vi "onStop.vi"(8 "error in (no error)":errorcluster, 11 "Client in":refnum<class "Client.lvclass">) -> (0 "error out":errorcluster, 3 "Client out":refnum<class "Client.lvclass">)   [LabVIEW 2013, in "MQTT Server.lvlib" / "Client.lvclass"]
uses:
  Client.lvclass
  MQTT_Base/MQTT_Base.lvclass
  Client.lvclass/Client.ctl
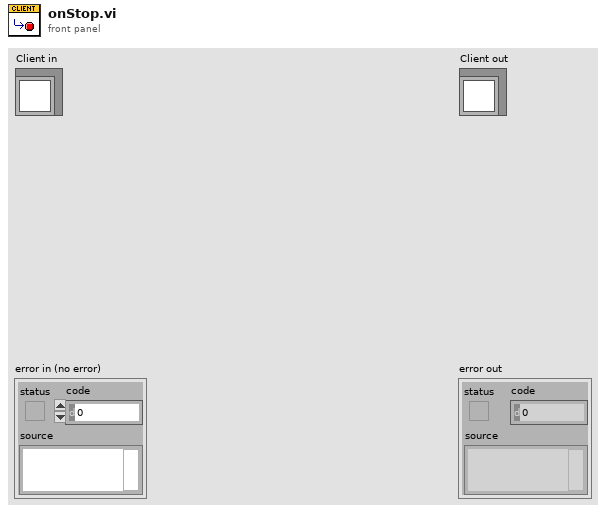
[diagram p1: front panel]
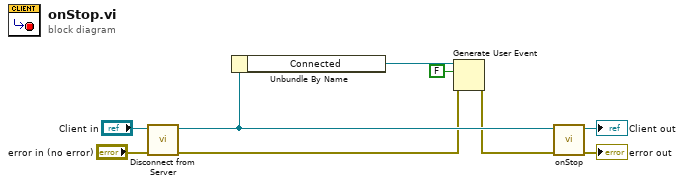
[diagram p0: block diagram]
diagram:
  n1 = call "Disconnect from Server.vi"("error in (no error)"="error in (no error)", "Client in"="Client in") -> ("error out"=w2:errorcluster, "Client out"=w5:refnum<class "Client.lvclass">)  [unwired: 8 in]
  n2 = Unbundle By Name(w5) -> ("Connected"=w4:refnum<user-event>)
  n3 = Generate User Event(user event=w4, event data cluster=FALSE ("event data"), error in=w2) -> (error out=w1:errorcluster)  [unwired: 1 in, 1 out]
  n4 = call-parent "onStop.vi"("error in (no error)"=w1, "MQTT_Base in"=w5) -> ("error out"=→"error out":errorcluster, "MQTT_Base out"=→"Client out":refnum<class "Client.lvclass">)  [unwired: 8 in]
